vi "Remove Engine Simulation Toolkit Custom Device.vi"(8 "error in (no error)":errorcluster, 11 "EST custom device in":refnum<k24>) -> (0 "error out":errorcluster)   [LabVIEW 2015, in "Engine Simulation Toolkit SysDef API.lvlib"]
uses:
  Engine Simulation Toolkit SysDef API.lvlib
  NationalInstruments.VeriStand.SystemDefinitionAPI
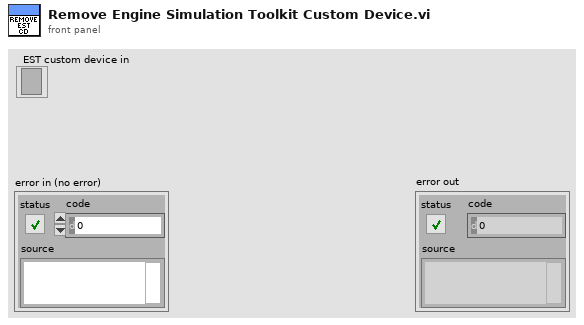
[diagram p1: front panel]
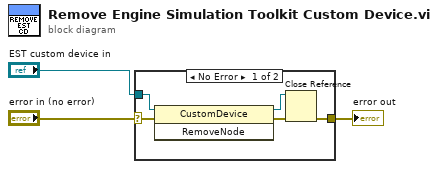
[diagram p0: block diagram]
diagram:
  n1 = case shown="No Error" "error in (no error)" {
    selector: "error in (no error)" -> [w5 w9]
    tunnel: "EST custom device in" -> [w4 _]
    tunnel: [w6 w9] -> w3
    frame No Error {
      n2 = invoke class="CustomDevice" method="RemoveNode"(reference=w4, error in=w5) -> (reference out=w8:refnum<k24>, error out=w7:errorcluster)  [unwired: 1 in, 1 out]
      n3 = Close Reference(reference=w8, error in (no error)=w7) -> (error out=w6:errorcluster)
    }
    frame Error {
    }
  }
  "error out" <- w3
